vi "Serial Read.vi"(8 "Error In":errorcluster, 10 "Bytes To Read":u32, 11 "LINX Device Config":T1) -> (0 "Error Out":errorcluster, 2 "Data":string, 3 "LINX Device Config":T1)   [LabVIEW 2011, in "LMH-LINX.lvlib" / "Device.lvlib"]
doc: "Read data from the serial port associated with the LINX device."
uses:
  Device.lvlib
  Type Defs/LINX Device Config.ctl
  Type Defs/Interface.ctl
  Type Defs/TCP Config.ctl
  Type Defs/Channels.ctl
  LMH-LINX.lvlib
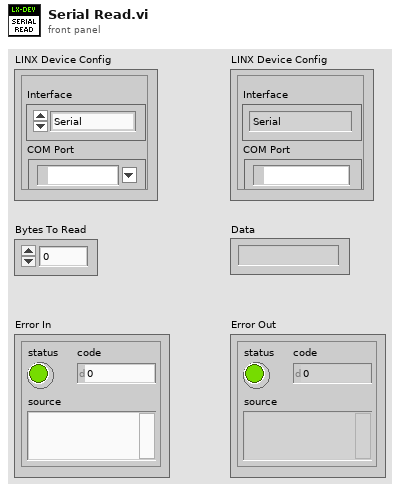
[diagram p1: front panel]
types:
  T1 = typedef "LMH-LINX.lvlib/Device.lvlib/LINX Device Config.ctl" = cluster{"Interface":T2, "COM Port":refnum<visa-resource-name>, "TCP Configuration":T3, "Device Family":u8, "Device ID":u8, "Device Name":string, "TCP Ref":refnum<k5>, "Channels":T4}
  T2 = typedef "LMH-LINX.lvlib/Interface.ctl" = enum16{"Serial", "TCP"}
  T3 = typedef "LMH-LINX.lvlib/Device.lvlib/TCP Config.ctl" = cluster{"IP Address":string, "Port":u16}
  T4 = typedef "LMH-LINX.lvlib/Channels.ctl" = cluster{"DI":u8[], "DO":u8[], "AI":u8[], "AO":u8[], "PWM":u8[], "QE":u8[], "UART":u8[], "I2C 2":u8[], "SPI":u8[], "CAN":u8[], "Servo":u8[], "AI Ref (V)":dbl, "AO Ref (V)":dbl, "AO Resolution (Bits)":u8}
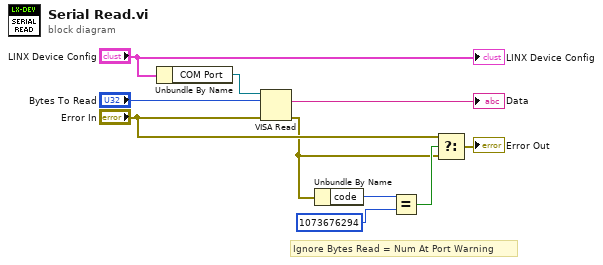
[diagram p0: block diagram]
diagram:
  # "Ignore Bytes Read = Num At Port Warning"
  n1 = Unbundle By Name("LINX Device Config") -> ("COM Port"=w9:refnum<visa-resource-name>)
  n2 = VISA Read(VISA resource name=w9, byte count="Bytes To Read", error in (no error)="Error In") -> (read buffer=→"Data":string, error out=w2:errorcluster)  [unwired: 2 out]
  n3 = Unbundle By Name(w2) -> ("code"=w6:i32)
  n4 = Equal?(x=w6, y=1073676294) -> (x = y?=w4:bool)
  n5 = Select(t="Error In", s=w4, f=w2) -> (s? t:f=→"Error Out":errorcluster)
  "LINX Device Config" <- "LINX Device Config"
